vi "TagMetadataToImage.vi"(8 "error in (no error)":errorcluster, 10 "Image In":T1, 11 "QPDController in":refnum<class "QPDController.lvclass">) -> (0 "error out":errorcluster, 2 "Image Out":T1, 3 "QPDController out":refnum<class "QPDController.lvclass">)   [LabVIEW 2020, in "QPDController.lvlib" / "QPDController.lvclass"]
uses:
  QPDController.lvclass
  <vilib>/vision/Image Controls.llb/IMAQ Image.ctl
  QPDController.lvclass/QPDController.ctl
  Model/Hardware Abstraction Layer/Component/GenericActor/GenericActor/GenericController.lvclass
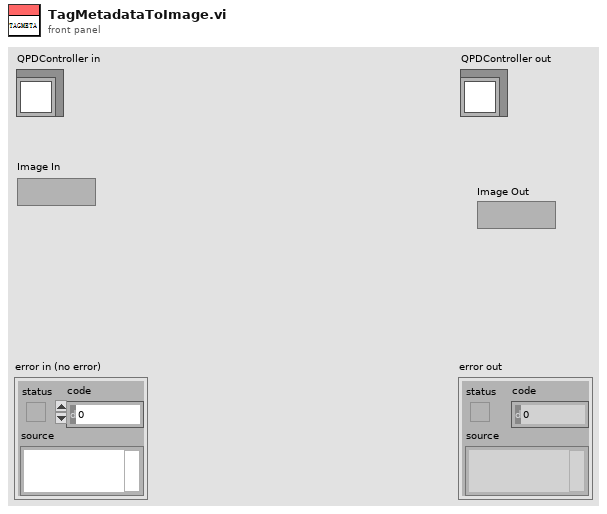
[diagram p1: front panel]
types:
  T1 = typedef "IMAQ Image.ctl" = refnum<image>
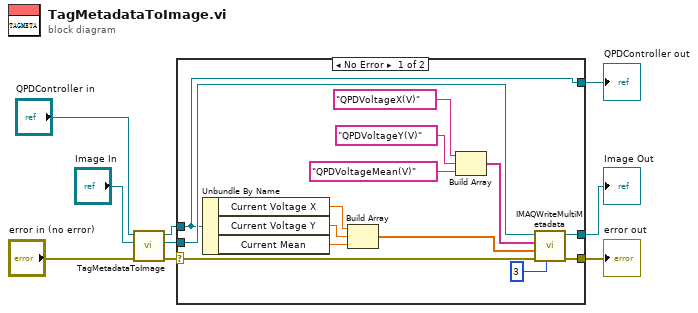
[diagram p0: block diagram]
diagram:
  n1 = call-parent "TagMetadataToImage.vi"("error in (no error)"="error in (no error)", "Image In"="Image In", "GenericController in"="QPDController in") -> ("error out"=w4:errorcluster, "Image Out"=w6:T1, "GenericController out"=w5:refnum<class "QPDController.lvclass">)  [unwired: 6 in]
  n2 = case shown="No Error" w4 {
    selector: w4 -> [w23 w26]
    tunnel: [w21 w26] -> w1
    tunnel: w6 -> [w22 w25]
    tunnel: [w20 w25] -> w3
    tunnel: [w10 w24] -> w2
    tunnel: w5 -> [w10 w24]
    frame No Error {
      n3 = Unbundle By Name(w10) -> ("Current Voltage X"=w15:dbl, "Current Voltage Y"=w14:dbl, "Current Mean"=w13:dbl)
      n4 = Build Array(w15, w14, w13) -> (w12:dbl[])
      n5 = Build Array("QPDVoltageX(V)" ("Key"), "QPDVoltageY(V)" ("Key"), "QPDVoltageMean(V)" ("Key")) -> (w16:string[])
      n6 = call "IMAQWriteMultiMetadata.vi"("precision (6)"=i16 3, "error in (no error)"=w23, "Values"=w12, "Keys"=w16, "Image In"=w22) -> ("error out"=w21:errorcluster, "Image Out"=w20:T1)  [unwired: 5 in]
    }
    frame Error {
    }
  }
  "error out" <- w1
  "QPDController out" <- w2
  "Image Out" <- w3
